vi "inverse_img.vi"(8 "error in (no error)":errorcluster, 11 "Image Src":T1) -> (0 "error out":errorcluster, 3 "Image Dst":T1)   [LabVIEW 2020]
uses:
  <vilib>/vision/Image Controls.llb/IMAQ Image.ctl
  c98cd7dc-d202-4aef-9647-32833259bf2e.vi
panel:
  in  "File Path":path
  in  "DebugOn?":bool
  out "Image Display":T1(plugin-control)
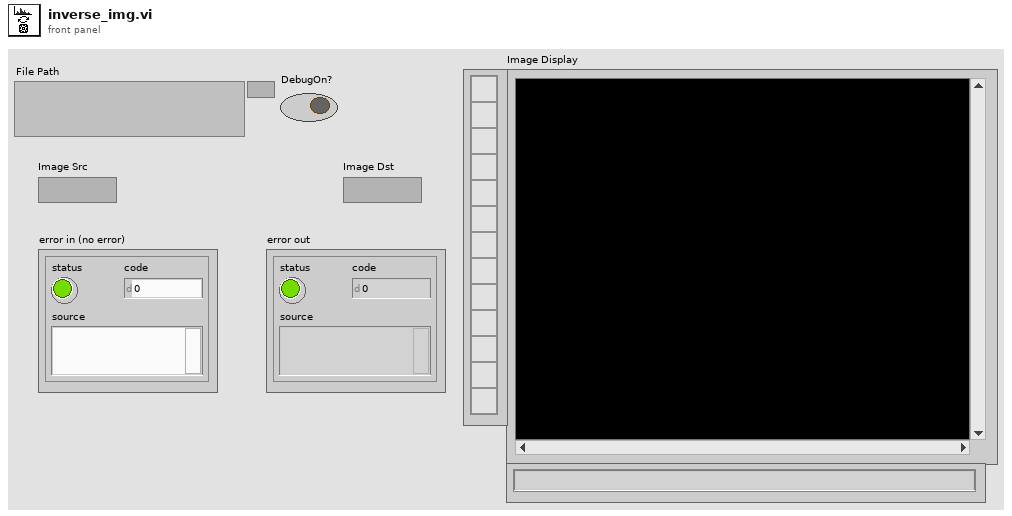
[diagram p1: front panel]
types:
  T1 = typedef "IMAQ Image.ctl" = refnum<image>
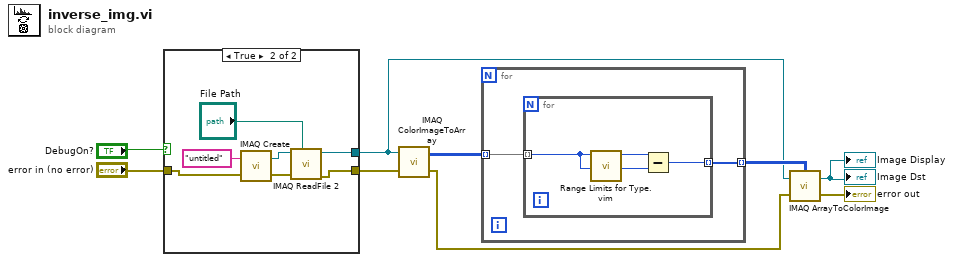
[diagram p0: block diagram]
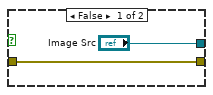
[diagram p2: hidden frame]
diagram:
  n1 = case shown="True" "DebugOn?" {
    tunnel: ["Image Src" w14] -> w1
    tunnel: [w10 w12] -> w5
    tunnel: "error in (no error)" -> [w10 w13]
    frame False {
    }
    frame True {
      n2 = call "IMAQ Create"("Image Name"="untitled", "error in (no error)"=w13) -> ("New Image"=w16:T1, "error out"=w17:errorcluster)  [unwired: 3 in]
      n3 = call "IMAQ ReadFile 2"("File Path"="File Path", "error in (no error)"=w17, "Image"=w16) -> ("error out"=w12:errorcluster, "Image Out"=w14:T1)  [unwired: 4 in, 3 out]
    }
  }
  n4 = call "IMAQ ColorImageToArray"("Image"=w1, "error in (no error)"=w5) -> ("Image Pixels (U32)"=w9:u32[][], "error out"=w3:errorcluster)  [unwired: 2 in, 1 out]
  n5 = for {
    tunnel: [w20] -> w8 mode=indexing
    tunnel: w9 -> [w19] mode=indexing
    n6 = for {
      tunnel: [w23] -> w20 mode=indexing
      tunnel: w19 -> [w21] mode=indexing
      n7 = call "Range Limits for Type.vim"("type"=w21) -> ("maximum value for type"=w22:u32)  [unwired: 9 in, 1 out]
      n8 = Subtract(x=w22, y=w21) -> (x-y=w23:u32)
    }
  }
  n9 = call "IMAQ ArrayToColorImage"("Image Pixels (U32)"=w8, "Image"=w1, "error in (no error)"=w3) -> ("Image Out"=→"Image Dst" →"Image Display":T1, "error out"=→"error out":errorcluster)  [unwired: 2 in]
